vi "Shut Down Device.vi"(8 "error in (no error)":errorcluster, 11 "Synchronization Device in":refnum<class "Synchronization Device.lvclass">) -> (0 "error out":errorcluster, 3 "Synchronization Device out":refnum<class "Synchronization Device.lvclass">)   [LabVIEW 2018, in "Synchronization Device.lvlib" / "Synchronization Device.lvclass"]
uses:
  Synchronization Device.lvclass
  Synchronization Device.lvclass/Synchronization Device.ctl
  <vilib>/DAQmx/write.llb/DAQmx Write (Digital 1D Bool 1Chan 1Samp).vi
  <vilib>/DAQmx/miscellaneous.llb/DAQmx Fill In Error Info.vi
  Device/Device.lvclass
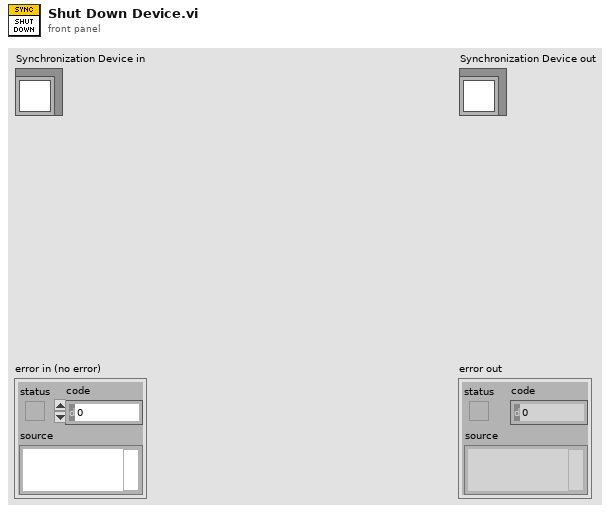
[diagram p1: front panel]
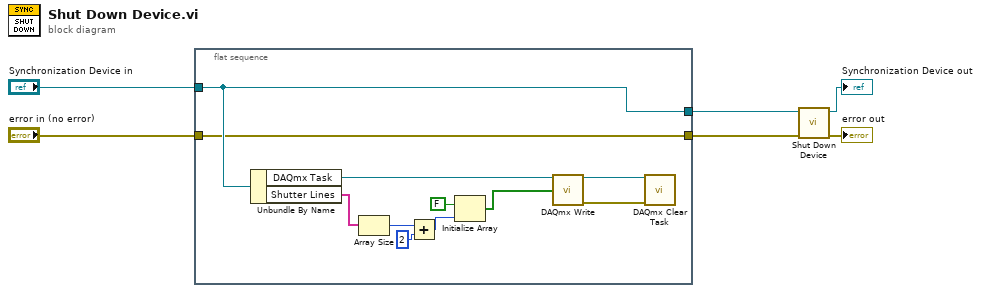
[diagram p0: block diagram]
diagram:
  n1 = flat-sequence {
    tunnel: "Synchronization Device in" -> [w12]
    tunnel: [w11] -> w3
    tunnel: [w12] -> w2
    tunnel: "error in (no error)" -> [w11]
    frame #0 {
      n2 = Unbundle By Name(w12) -> ("DAQmx Task"=w8:refnum<k21>, "Shutter Lines"=w7:string[])
      n3 = Array Size(array=w7) -> (size(s)=w17:i32)
      n4 = Add(x=w17, y=2) -> (x+y=w14:i32)
      n5 = Initialize Array(FALSE ("element"), w14) -> (w13:bool[])
      n6 = call-poly <vilib>:"DAQmx Write.vi"("task/channels in"=w8, "data"=w13) -> ("task out"=w10:refnum<k21>, "error out"=w9:errorcluster)  [unwired: 11 in, 1 out]
      n7 = call <vilib>:"DAQmx Clear Task.vi"("task in"=w10, "error in"=w9) -> ()  [unwired: 13 in, 1 out]
    }
  }
  n8 = call-parent "Shut Down Device.vi"("error in (no error)"=w3, "Device in"=w2) -> ("error out"=→"error out":errorcluster, "Device out"=→"Synchronization Device out":refnum<class "Synchronization Device.lvclass">)  [unwired: 8 in]
